vi "Two Path Dummy.vi"(8 "error in (no error)":errorcluster, 11 "Boolean":bool) -> (0 "error out":errorcluster)   [LabVIEW 2020]
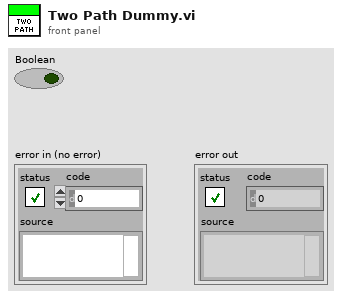
[diagram p1: front panel]
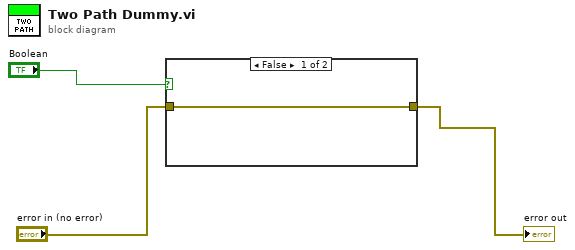
[diagram p0: block diagram]
diagram:
  n1 = case shown="False" "Boolean" {
    tunnel: [w4 w5] -> w1
    tunnel: "error in (no error)" -> [w4 w5]
    frame False {
    }
    frame True {
    }
  }
  "error out" <- w1
